vi "Index uebersetzen.vi"(6 "Aktion":T3, 11 "Array":i32[][](array[numeric])) -> (2 "Komponenten":i32[](array[numeric]), 3 "Komponenten":T1 caption="Cluster")   [LabVIEW 2020, in "EPA 1065.lvlib" / "Interference verificaton 1065-366.lvlib"]
uses:
  Interference verificaton 1065-366.lvlib
  Aktion Index uebersetzten.ctl
  Komponenten.ctl
  Visualisierungs Elemente/String - Ausgabefeld.ctl
  Seiten/FT-IR/FGV FT-IR Gasliste Aktionen.ctl
  Aktion FGV Interference.ctl
  Seiten/FT-IR/FT-IR.lvlib
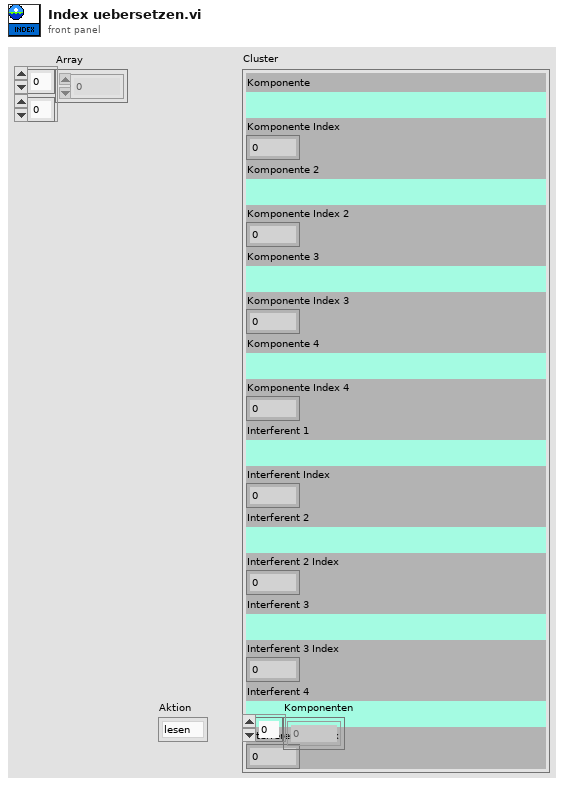
[diagram p1: front panel]
types:
  T1 = typedef "EPA 1065.lvlib/Interference verificaton 1065-366.lvlib/Komponenten.ctl" = cluster{"Komponente":T2, "Komponente Index":i32, "Komponente 2":T2, "Komponente Index 2":i32, "Komponente 3":T2, "Komponente Index 3":i32, "Komponente 4":T2, "Komponente Index 4":i32, "Interferent 1":T2, "Interferent Index":i32, "Interferent 2":T2, "Interferent 2 Index":i32, "Interferent 3":T2, "Interferent 3 Index":i32, "Interferent 4":T2, "Interferent 4 Index":i32}
  T2 = typedef "String - Ausgabefeld.ctl" = string
  T3 = typedef "EPA 1065.lvlib/Interference verificaton 1065-366.lvlib/Aktion Index uebersetzten.ctl" = enum16{"lesen", "schreiben", "auswerten"}
  T4 = typedef "EPA 1065.lvlib/Interference verificaton 1065-366.lvlib/Aktion FGV Interference.ctl" = enum16{"Lesen", "TestKonfig", "TestSetting", "Einheiten", "Ergebnis", "Laden", "Tabelle", "Speichern", "löschen"}
  T5 = typedef "FT-IR.lvlib/FGV FT-IR Gasliste Aktionen.ctl" = enum16{"lesen", "Gasliste FT-IR", "Gasliste ausgelesen", "laden", "speichern", "löschen"}
  T6 = typedef "EPA 1065.lvlib/Interference verificaton 1065-366.lvlib/TestKonfig.ctl" = cluster{"CH4:":u16, "Ethane:":u16, "NMHC:":u16, "NMNEHC:":u16, "Komp 1 aktiv:":bool, "Komp 2 aktiv:":bool, "Komp 3 aktiv:":bool, "Komp 4 aktiv:":bool, "Modus":T7, "CG Aufschaltzeit:":dbl, "Interferent 1: CO2":u16, "Interferent 2: H2O":u16, "Interferent 3: CH4":u16, "Interferent 4: C2H6 / C3H8":u16, "Gasflaschen Nr.:":string, "Gasflaschen Nr.: 3":string, "Gasflaschen Nr.: 4":string, "Inter 1 aktiv":bool, "Inter 2 aktiv":bool, "Inter 3 aktiv":bool, "Inter 4 aktiv":bool, "Accuracy":string, "Accuracy 3":string, "Accuracy 4":string, "Konzentration 1:":dbl, "Konzentration 2:":dbl, "Konzentration 3:":dbl, "Konzentration 4:":dbl, "Flow weighted mean 1:":dbl, "Flow weighted mean 2:":dbl, "Flow weighted mean 3:":dbl, "Flow weighted mean 4:":dbl}
  T7 = typedef "EPA 1065.lvlib/Interference verificaton 1065-366.lvlib/Modus.ctl" = u16
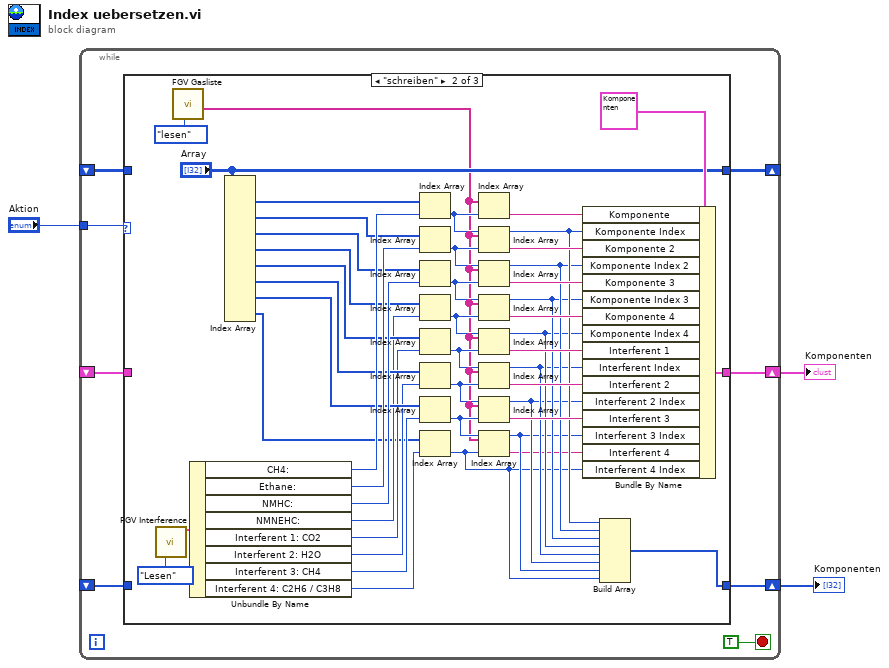
[diagram p0: block diagram]
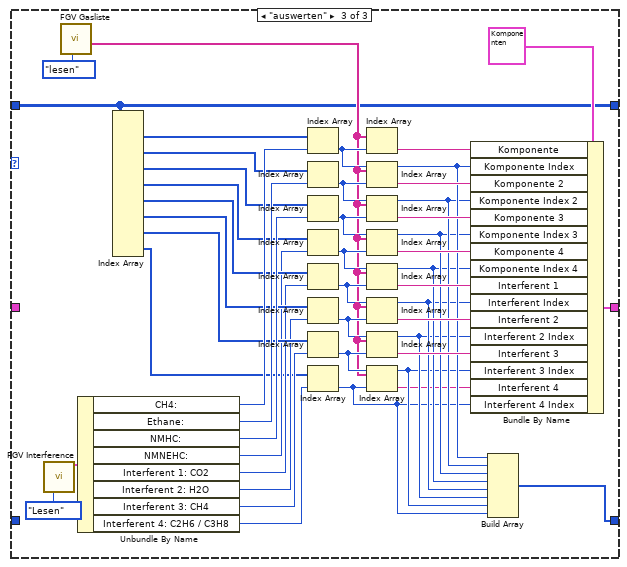
[diagram p3: hidden frame]
diagram:
  n1 = while {
    tunnel: "Aktion" -> [w10]
    shift-right: [w9] -> w2
    shift-left: _ -> [w8]
    shift-right: [w7] -> _
    shift-left: _ -> [w6]
    shift-right: [w5] -> w1
    shift-left: _ -> [w4]
    stop <- TRUE stop-if-true
    n2 = case shown="\"schreiben\"" w10 {
      tunnel: [w14 w49 w89] -> w9
      tunnel: w8 -> [w14 _ _]
      tunnel: [w12 "Array" w55] -> w7
      tunnel: w6 -> [w12 _ w55]
      tunnel: [w13 w24 w65] -> w5
      tunnel: w4 -> [w13 _ _]
      frame "lesen", Default {
      }
      frame "schreiben" {
        n3 = call "FGV Interference.vi"("Aktion FGV Interference"=Aktion_FGV_Interference."Lesen") -> ("TestKonfig"=w53:T6)  [unwired: 9 in, 5 out]
        n4 = call "FGV Gasliste.vi"("Aktionen"=FGV_FT-IR_Gasliste_Aktionen."lesen") -> ("Aktuelle Gasliste gesamt"=w17:T2[])  [unwired: 8 in, 2 out]
        n5 = Unbundle By Name(w53) -> ("CH4:"=w46:u16, "Ethane:"=w47:u16, "NMHC:"=w54:u16, "NMNEHC:"=w23:u16, "Interferent 1: CO2"=w22:u16, "Interferent 2: H2O"=w21:u16, "Interferent 3: CH4"=w20:u16, "Interferent 4: C2H6 / C3H8"=w18:u16)
        n6 = Index Array(array="Array") -> (element #1=w45:i32[], element #2=w43:i32[], element #3=w40:i32[], element #4=w38:i32[], element #5=w36:i32[], element #6=w34:i32[], element #7=w32:i32[], element #8=w19:i32[])  [unwired: 16 in]
        n7 = Index Array(array=w45, index=w46) -> (element=w31:i32)
        n8 = Index Array(array=w43, index=w47) -> (element=w30:i32)
        n9 = Index Array(array=w40, index=w54) -> (element=w29:i32)
        n10 = Index Array(array=w38, index=w23) -> (element=w28:i32)
        n11 = Index Array(array=w36, index=w22) -> (element=w27:i32)
        n12 = Index Array(array=w34, index=w21) -> (element=w26:i32)
        n13 = Index Array(array=w32, index=w20) -> (element=w25:i32)
        n14 = Index Array(array=w19, index=w18) -> (element=w15:i32)
        n15 = Index Array(array=w17, index=w31) -> (element=w44:T2)
        n16 = Index Array(array=w17, index=w30) -> (element=w42:T2)
        n17 = Index Array(array=w17, index=w29) -> (element=w41:T2)
        n18 = Index Array(array=w17, index=w28) -> (element=w39:T2)
        n19 = Index Array(array=w17, index=w27) -> (element=w37:T2)
        n20 = Index Array(array=w17, index=w26) -> (element=w35:T2)
        n21 = Index Array(array=w17, index=w25) -> (element=w33:T2)
        n22 = Index Array(array=w17, index=w15) -> (element=w16:T2)
        n23 = Bundle By Name(cluster=T1 {"Komponente"="", "Komponente Index"=0, "Komponente 2"="", "Komponente Index 2"=0, "Komponente 3"="", "Komponente Index 3"=0, "Komponente 4"="", "Komponente Index 4"=0, "Interferent 1"="", "Interferent Index"=0, "Interferent 2"="", "Interferent 2 Index"=0, "Interferent 3"="", "Interferent 3 Index"=0, "Interferent 4"="", "Interferent 4 Index"=0} ("Komponenten"), "Komponente"=w44, "Komponente Index"=w31, "Komponente 2"=w42, "Komponente Index 2"=w30, "Komponente 3"=w41, "Komponente Index 3"=w29, "Komponente 4"=w39, "Komponente Index 4"=w28, "Interferent 1"=w37, "Interferent Index"=w27, "Interferent 2"=w35, "Interferent 2 Index"=w26, "Interferent 3"=w33, "Interferent 3 Index"=w25, "Interferent 4"=w16, "Interferent 4 Index"=w15) -> (w49:T1)
        n24 = Build Array(w31, w30, w29, w28, w27, w26, w25, w15) -> (w24:i32[])
      }
      frame "auswerten" {
        n25 = call "FGV Interference.vi"("Aktion FGV Interference"=Aktion_FGV_Interference."Lesen") -> ("TestKonfig"=w93:T6)  [unwired: 9 in, 5 out]
        n26 = call "FGV Gasliste.vi"("Aktionen"=FGV_FT-IR_Gasliste_Aktionen."lesen") -> ("Aktuelle Gasliste gesamt"=w58:T2[])  [unwired: 8 in, 2 out]
        n27 = Unbundle By Name(w93) -> ("CH4:"=w87:u16, "Ethane:"=w88:u16, "NMHC:"=w94:u16, "NMNEHC:"=w64:u16, "Interferent 1: CO2"=w63:u16, "Interferent 2: H2O"=w62:u16, "Interferent 3: CH4"=w61:u16, "Interferent 4: C2H6 / C3H8"=w59:u16)
        n28 = Index Array(array=w55) -> (element #1=w86:i32[], element #2=w84:i32[], element #3=w81:i32[], element #4=w79:i32[], element #5=w77:i32[], element #6=w75:i32[], element #7=w73:i32[], element #8=w60:i32[])  [unwired: 16 in]
        n29 = Index Array(array=w86, index=w87) -> (element=w72:i32)
        n30 = Index Array(array=w84, index=w88) -> (element=w71:i32)
        n31 = Index Array(array=w81, index=w94) -> (element=w70:i32)
        n32 = Index Array(array=w79, index=w64) -> (element=w69:i32)
        n33 = Index Array(array=w77, index=w63) -> (element=w68:i32)
        n34 = Index Array(array=w75, index=w62) -> (element=w67:i32)
        n35 = Index Array(array=w73, index=w61) -> (element=w66:i32)
        n36 = Index Array(array=w60, index=w59) -> (element=w56:i32)
        n37 = Index Array(array=w58, index=w72) -> (element=w85:T2)
        n38 = Index Array(array=w58, index=w71) -> (element=w83:T2)
        n39 = Index Array(array=w58, index=w70) -> (element=w82:T2)
        n40 = Index Array(array=w58, index=w69) -> (element=w80:T2)
        n41 = Index Array(array=w58, index=w68) -> (element=w78:T2)
        n42 = Index Array(array=w58, index=w67) -> (element=w76:T2)
        n43 = Index Array(array=w58, index=w66) -> (element=w74:T2)
        n44 = Index Array(array=w58, index=w56) -> (element=w57:T2)
        n45 = Bundle By Name(cluster=T1 {"Komponente"="", "Komponente Index"=0, "Komponente 2"="", "Komponente Index 2"=0, "Komponente 3"="", "Komponente Index 3"=0, "Komponente 4"="", "Komponente Index 4"=0, "Interferent 1"="", "Interferent Index"=0, "Interferent 2"="", "Interferent 2 Index"=0, "Interferent 3"="", "Interferent 3 Index"=0, "Interferent 4"="", "Interferent 4 Index"=0} ("Komponenten"), "Komponente"=w85, "Komponente Index"=w72, "Komponente 2"=w83, "Komponente Index 2"=w71, "Komponente 3"=w82, "Komponente Index 3"=w70, "Komponente 4"=w80, "Komponente Index 4"=w69, "Interferent 1"=w78, "Interferent Index"=w68, "Interferent 2"=w76, "Interferent 2 Index"=w67, "Interferent 3"=w74, "Interferent 3 Index"=w66, "Interferent 4"=w57, "Interferent 4 Index"=w56) -> (w89:T1)
        n46 = Build Array(w72, w71, w70, w69, w68, w67, w66, w56) -> (w65:i32[])
      }
    }
  }
  "Komponenten" <- w2
  "Komponenten" <- w1
